vi "configure.vi"(8 "error in (no error)":errorcluster, 11 "Hardware in":refnum<class "Hardware.lvclass">) -> (0 "error out":errorcluster, 3 "Hardware out":refnum<class "Hardware.lvclass">)   [LabVIEW 2017, in "Hardware.lvlib" / "Hardware.lvclass"]
uses:
  Hardware.lvclass
  HW Config/HW Configuration.lvclass/HW Configuration.ctl
  Hardware.lvclass/Hardware.ctl
  HW Config/Read IO Mapping.vi
  HW Config/HW Configuration.lvclass
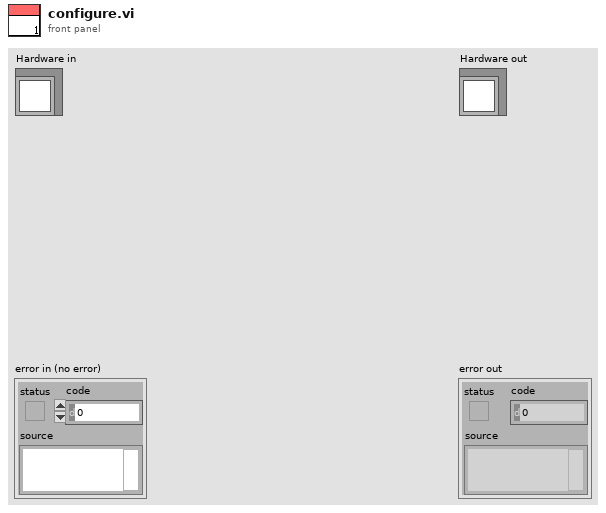
[diagram p1: front panel]
types:
  T1 = cluster{"Device Name":string, "Channel Mapping (Device -> Channel)":string[][]}
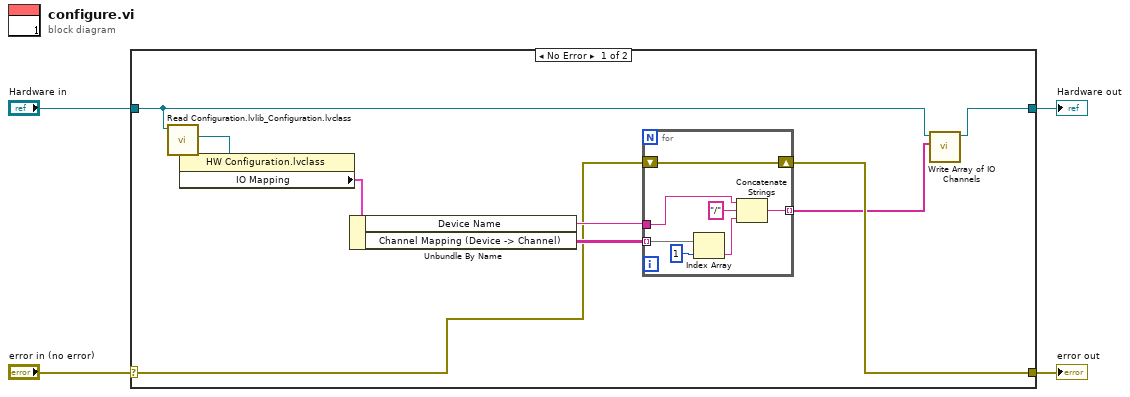
[diagram p0: block diagram]
diagram:
  n1 = case shown="No Error" "error in (no error)" {
    selector: "error in (no error)" -> [w9 w22]
    tunnel: [w8 w22] -> w3
    tunnel: [w5 w21] -> w1
    tunnel: "Hardware in" -> [w6 w21]
    frame No Error {
      n2 = call-dynamic "Read Configuration.lvlib_Configuration.lvclass.vi"("Hardware in"=w6) -> ("Hardware.lvlib:HW Configuration.lvclass"=w13:refnum<class "HW Configuration.lvclass">)  [unwired: 8 in, 2 out]
      n3 = property class="HW Configuration.lvclass"(reference=w13) -> ("IO Mapping"=w12:T1)  [unwired: 1 in, 2 out]
      n4 = Unbundle By Name(w12) -> ("Device Name"=w10:string, "Channel Mapping (Device -> Channel)"=w11:string[][])
      n5 = for {
        tunnel: w11 -> [w20] mode=indexing
        shift-right: [w19] -> w8
        shift-left: w9 -> [w19]
        tunnel: [w16] -> w7 mode=indexing
        tunnel: w10 -> [w15]
        n6 = Index Array(array=w20, index=1) -> (element=w17:string)
        n7 = Concatenate Strings(w15, "/" ("string"), w17) -> (w16:string)
      }
      n8 = call "Write Array of IO Channels.vi"("Array of IO Channels"=w7, "Hardware in"=w6) -> ("Hardware out"=w5:refnum<class "Hardware.lvclass">)  [unwired: 8 in, 1 out]
    }
    frame Error {
    }
  }
  "error out" <- w3
  "Hardware out" <- w1
